vi "Mapping v10.4.0.vi"(5 "Simulate Spectra":bool, 7 "Simulate Drive":bool, 11 "Input Parameters":T9={"CCD3000 Connection"={"Comm Interface"=1, "BUS"=0, "Address"=5, "Com Port"=1}, "Drive Connection Settings"={"Objective GPIB-Port"=4, "Stage GPIB-Port"=4, "Drive Selector"=0, "Drive Velocity (V/s)"=5.0}, "ITC503 Current Values"={"ITC503 Heater"=0.0, "ITC503 Temperature"=0.0, "ITC503 P"=0.0, "ITC503 I"=0.0, "ITC503 D"=0.0, "ITC503 Setpoint"=0.0, "ITC503 Gradient"=0.0, "ITC503 Heater Auto"=FALSE, "ITC503 PID Auto"=FALSE}, "Wavelengths (nm)"=[], "Drive Current Values"={"Voltages"={"Drive X Voltage"=0.0, "Drive Y Voltage"=0.0, "Drive Z Voltage"=0.0}, "Position"={"Drive X Position"=0.0, "Drive Y Position"=0.0, "Drive Z Position"=0.0}}, "iHR Current Values"={"iHR 550 Front Entrance"=0.0, "iHR550 Side Exit"=0.0, "iHR550 Wavelength"=897.9988, "iHR550 Exit Mirror"=2, "iHR550 Grating"="1", "Grating Index"=1}, "Spectra Settings"={"Integration Time"=1.0, "Repetitions"=1, "Mapping Spectra"=TRUE}, "CCD3500 Temperature"=0.0, "Simulate Drive"=FALSE, "Simulate Spectra"=FALSE} {"CCD3500 Temperature" min=10.0 max=160.0 step=0.1 format="%.1f"; "Spectra Settings"."Repetitions" min=1 max=100 step=1; "Spectra Settings"."Integration Time" min=0.5 max=6000.0 step=1.0 format="%.1f"; "iHR Current Values"."iHR550 Exit Mirror" items=["EntranceMirror", "ExitMirror", "Front", "Side"]; "Drive Current Values"."Position"."Drive Z Position" min=-273.0 max=300000.0 step=0.0001 format="%.1f"; "Drive Current Values"."Position"."Drive Y Position" min=-273.0 max=300000.0 step=0.0001 format="%.1f"; "Drive Current Values"."Position"."Drive X Position" min=-273.0 max=300000.0 step=0.0001 format="%.1f"; "Drive Current Values"."Voltages"."Drive Z Voltage" min=-273.0 max=300000.0 step=0.0001 format="%.1f"; "Drive Current Values"."Voltages"."Drive Y Voltage" min=-273.0 max=300000.0 step=0.0001 format="%.1f"; "Drive Current Values"."Voltages"."Drive X Voltage" min=-273.0 max=300000.0 step=0.0001 format="%.1f"; "ITC503 Current Values"."ITC503 Gradient" format="%.2f"; "ITC503 Current Values"."ITC503 Setpoint" min=-273.0 max=300000.0 step=0.0001 format="%.1f"; "ITC503 Current Values"."ITC503 I" format="%_1f"; "ITC503 Current Values"."ITC503 P" format="%_1f"; "ITC503 Current Values"."ITC503 Temperature" min=0.0 max=1645.0 step=1e-05 format="%.2f"; "ITC503 Current Values"."ITC503 Heater" min=0.0 max=100.0 step=0.01 scale=0.0..100.0; "Drive Connection Settings"."Drive Velocity (V/s)" min=10.0 max=160.0 step=0.1 format="%.1f"; "Drive Connection Settings"."Drive Selector" items=["Obj.", "Stage"]; "Drive Connection Settings"."Stage GPIB-Port" min=1 max=20 step=1 format="%#.0f"; "Drive Connection Settings"."Objective GPIB-Port" min=1 max=20 step=1 format="%#.0f"; "CCD3000 Connection"."Comm Interface" items=["RS 232", "GPIB"]}) -> ()   [LabVIEW 2010]
uses:
  ESA-C/TypeDefs/ESA-C Connection Settings.ctl
  TypeDefs/Mapping Spectra Params.ctl
  TypeDefs/Mapping Drive Params.ctl
  ESA-C/TypeDefs/ESA-C Set Positions.ctl
  ESA-C/TypeDefs/ESA-C Current Values.ctl
  iHR550/TypeDefs/iHR Current Values.ctl
  ITC503/TypeDefs/ITC503 Current Values.ctl
  drivers/Horiba Spectrum One 3000V/Lib/CCD_command.llb/Comm Params.ctl
  <vilib>/Utility/miscctls.llb/LVPointTypeDef.ctl
  Global Variables.vi
panel:
  out "AutoClose":bool
  out "ITC503 Temperature":dbl caption="Sample (K)" min=10.0 max=160.0 step=0.1 format="%.1f"
  out "CCD3500 Temperature":dbl caption="CCD (°C)" min=10.0 max=160.0 step=0.1 format="%.1f"
  in  "CCD3000 Current Rep.":string="0/0"
  in  "Pause":bool
  out "Current Position":T1 {"Position"."Drive Z Position" min=-273.0 max=300000.0 step=0.0001 format="%.1f"; "Position"."Drive Y Position" min=-273.0 max=300000.0 step=0.0001 format="%.1f"; "Position"."Drive X Position" min=-273.0 max=300000.0 step=0.0001 format="%.1f"; "Voltages"."Drive Z Voltage" min=-273.0 max=300000.0 step=0.0001 format="%.1f"; "Voltages"."Drive Y Voltage" min=-273.0 max=300000.0 step=0.0001 format="%.1f"; "Voltages"."Drive X Voltage" min=-273.0 max=300000.0 step=0.0001 format="%.1f"}
  out "Target Position":T2={"Drive X Set"=10.0, "Drive Y Set"=10.0, "Drive Z Set"=10.0} {"Drive X Set" min=10.0 max=160.0 step=0.1 format="%.1f"; "Drive Z Set" min=10.0 max=160.0 step=0.1 format="%.1f"; "Drive Y Set" min=10.0 max=160.0 step=0.1 format="%.1f"}
  out "Progress":u8(slide) max=10 scale=0.0..100.0
  out "Objective Running":bool caption="Obj."
  out "CCD Running":bool caption="CCD"
  in  "Save Map":bool
  in  "Spectra Params":T3={"Integration Time"=10.0, "Repetitions"=10, "Mapping Spectra"=TRUE} {"Repetitions" min=1 max=100 step=1; "Integration Time" min=0.5 max=6000.0 step=1.0 format="%.1f"}
  in  "Drive Settings":T4={"Objective GPIB-Port"=4, "Stage GPIB-Port"=4, "Drive Selector"=0, "Drive Velocity (V/s)"=5.0} {"Drive Velocity (V/s)" min=10.0 max=160.0 step=0.1 format="%.1f"; "Drive Selector" items=["Obj.", "Stage"]; "Stage GPIB-Port" min=1 max=20 step=1 format="%#.0f"; "Objective GPIB-Port" min=1 max=20 step=1 format="%#.0f"}
  in  "Z Position":dbl caption="Z (µm)" min=0.0 max=100.0 step=0.1 format="%.1f"
  in  "Mapping Params":T5={"X Start Position"=0.0, "X Stop Position"=10.0, "Y Start Position"=0.0, "Y Stop Position"=10.0, "Step Size"=1.0} {"Step Size" min=0.1 max=30.0 step=0.1 format="%.1f"; "Y Stop Position" min=0.0 max=30.0 step=0.1 format="%.1f"; "Y Start Position" min=0.0 max=30.0 step=0.1 format="%.1f"; "X Stop Position" min=0.0 max=30.0 step=0.1 format="%.1f"; "X Start Position" min=0.0 max=30.0 step=0.1 format="%.1f"}
  in  "Exit":bool
  out "Measuring":bool
  in  "Start":bool
  out "Filename":string
  out "Full Data":dbl[][](array[numeric])
  in  "CCD3500V Connection":T10={"Comm Interface"=1, "BUS"=0, "Address"=5, "Com Port"=0}
  out "Live Data":dbl[][](array[numeric])
  in  "ITC503 Current Values":T7 {"ITC503 Gradient" format="%.2f"; "ITC503 Setpoint" min=-273.0 max=300000.0 step=0.0001 format="%.1f"; "ITC503 I" format="%_1f"; "ITC503 P" format="%_1f"; "ITC503 Temperature" min=0.0 max=1645.0 step=1e-05 format="%.2f"; "ITC503 Heater" min=0.0 max=100.0 step=0.01 scale=0.0..100.0}
  in  "iHR Current Values":T8={"iHR 550 Front Entrance"=0.0, "iHR550 Side Exit"=0.0, "iHR550 Wavelength"=897.9988, "iHR550 Exit Mirror"=2, "iHR550 Grating"="1", "Grating Index"=1} {"iHR550 Exit Mirror" items=["EntranceMirror", "ExitMirror", "Front", "Side"]}
  in  "Wavelengths (nm)":dbl[](array[numeric])
  # "Status"
  # "Active"
  # "Target"
  # "Current"
  # "Parameters"
  # "Spectral"
  # "Spectral / Video Mapping"
  # "Mapping"
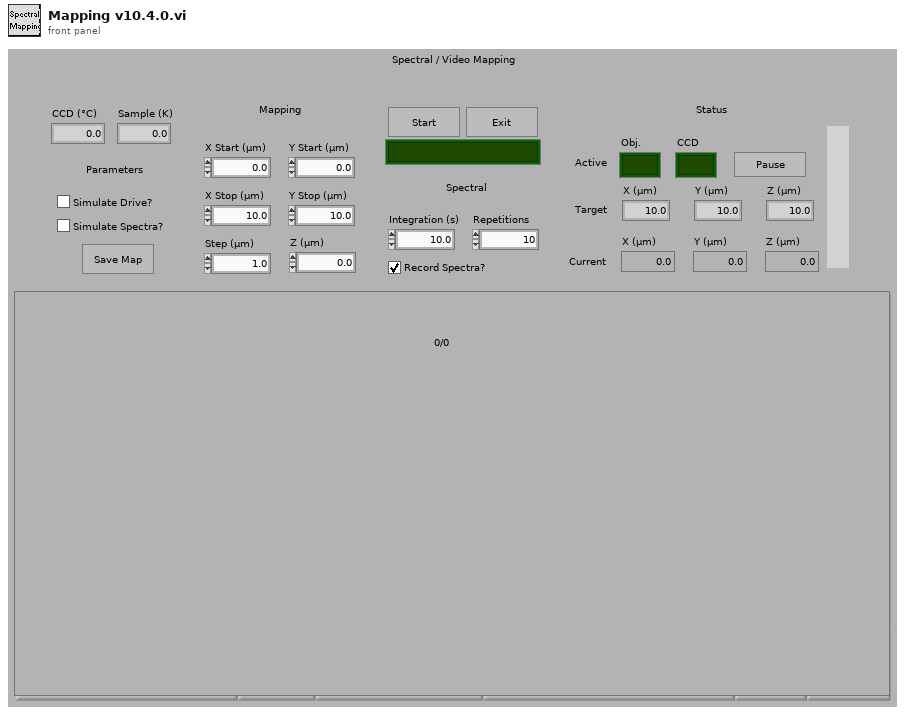
[diagram p1: front panel]
types:
  T1 = typedef "ESA-C Current Values.ctl" = cluster{"Voltages":cluster{"Drive X Voltage":dbl, "Drive Y Voltage":dbl, "Drive Z Voltage":dbl}, "Position":cluster{"Drive X Position":dbl, "Drive Y Position":dbl, "Drive Z Position":dbl}}
  T2 = typedef "ESA-C Set Positions.ctl" = cluster{"Drive X Set":dbl, "Drive Y Set":dbl, "Drive Z Set":dbl}
  T3 = typedef "Mapping Spectra Params.ctl" = cluster{"Integration Time":dbl, "Repetitions":u16, "Mapping Spectra":bool}
  T4 = typedef "ESA-C Connection Settings.ctl" = cluster{"Objective GPIB-Port":i32, "Stage GPIB-Port":i32, "Drive Selector":u16, "Drive Velocity (V/s)":dbl}
  T5 = typedef "Mapping Drive Params.ctl" = cluster{"X Start Position":dbl, "X Stop Position":dbl, "Y Start Position":dbl, "Y Stop Position":dbl, "Step Size":dbl}
  T6 = typedef "Comm Params.ctl" = cluster{"Comm Interface":u16, "BUS":i16, "Address":i16, "Com Port":i32}
  T7 = typedef "ITC503 Current Values.ctl" = cluster{"ITC503 Heater":dbl, "ITC503 Temperature":dbl, "ITC503 P":dbl, "ITC503 I":dbl, "ITC503 D":dbl, "ITC503 Setpoint":dbl, "ITC503 Gradient":dbl, "ITC503 Heater Auto":bool, "ITC503 PID Auto":bool}
  T8 = typedef "iHR Current Values.ctl" = cluster{"iHR 550 Front Entrance":dbl, "iHR550 Side Exit":dbl, "iHR550 Wavelength":dbl, "iHR550 Exit Mirror":i32, "iHR550 Grating":string, "Grating Index":i32}
  T9 = cluster{"CCD3000 Connection":T6, "Drive Connection Settings":T4, "ITC503 Current Values":T7, "Wavelengths (nm)":dbl[], "Drive Current Values":T1, "iHR Current Values":T8, "Spectra Settings":T3, "CCD3500 Temperature":dbl, "Simulate Drive":bool, "Simulate Spectra":bool}
  T10 = cluster{"Comm Interface":u16, "BUS":i16, "Address":i16, "Com Port":i32}
  T11 = cluster{"CCD3000 Connection":T6, "Drive Connection Settings":T4, "ITC503 Current Values":T7, "Wavelengths (nm)":dbl[], "Drive Current Values":T1, "iHR Current Values":T8, "Spectra Settings":T3, "CCD3500 Temperature":dbl, "Simulate Drive 2":bool, "Simulate Spectra 2":bool}
  T12 = typedef "LVPointTypeDef.ctl" = cluster{"Horizontal":i16, "Vertical":i16}
  T13 = typedef "NPC3SG Set Positions.ctl" = cluster{"Drive X Set":dbl, "Drive Y Set":dbl, "Drive Z Set":dbl}
  T14 = cluster{"Intensities":dbl[], "Wavelengths":dbl[]}[]
  T15 = cluster{"Intensities":dbl[], "Wavelengths":dbl[]}
  T16 = enum32{"invalid app kind", "Development System", "Run Time System", "Student Edition", "Embedded LabVIEW", "Evaluation", "Custom"}
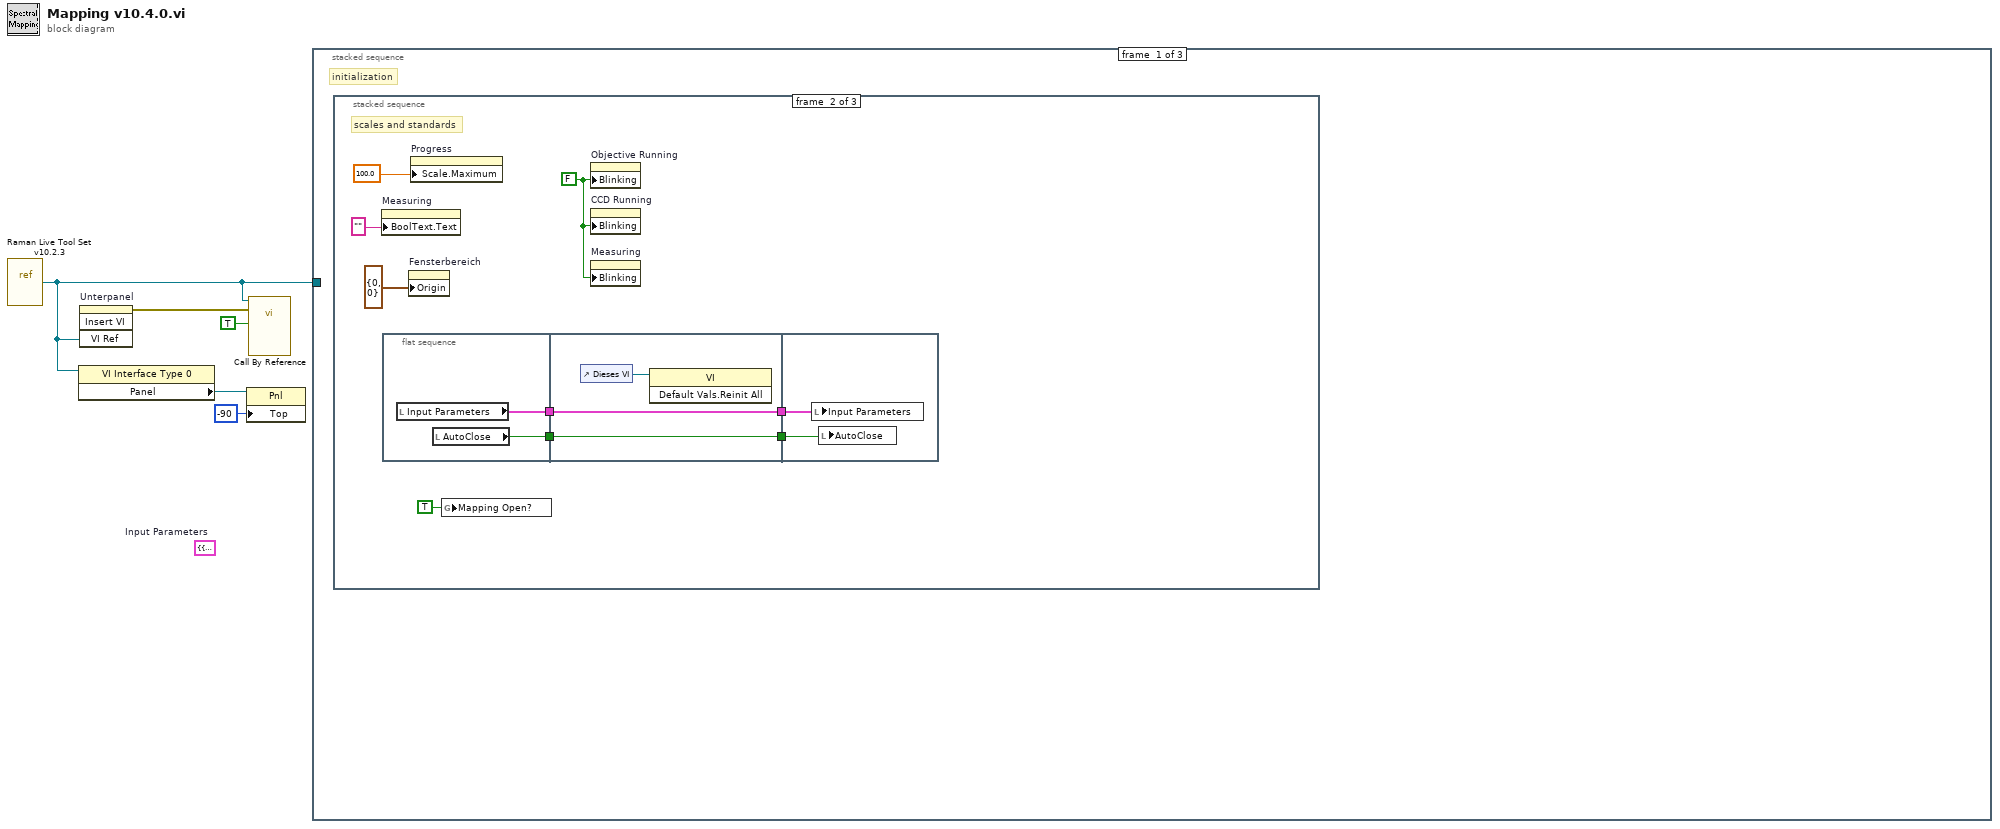
[diagram p0: block diagram]
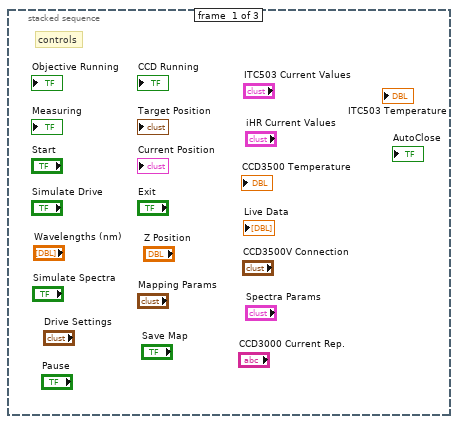
[diagram p2: hidden frame]
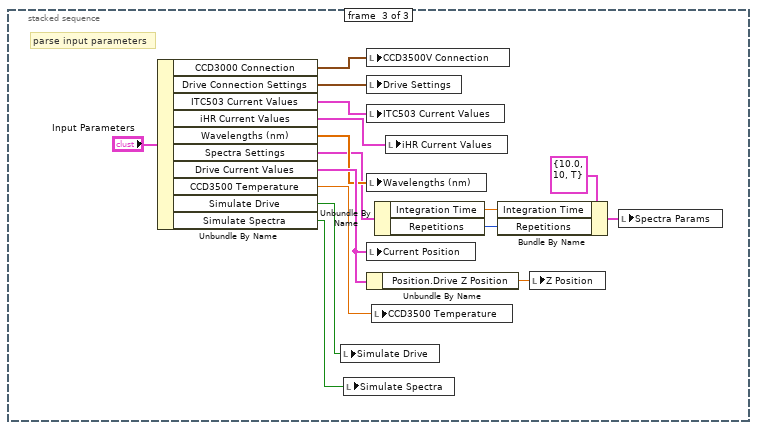
[diagram p3: hidden frame]
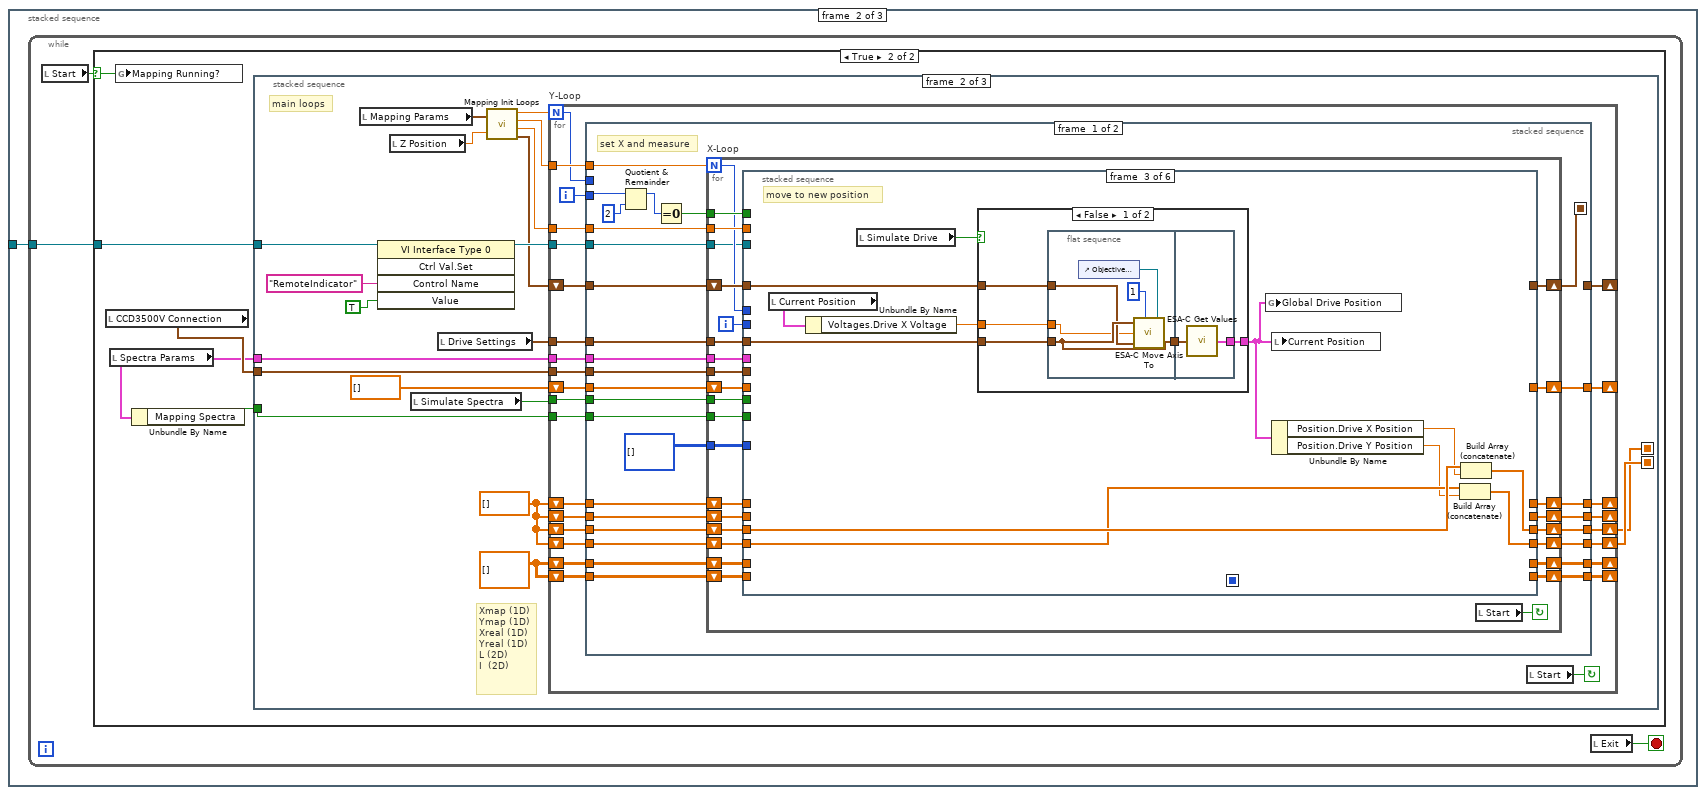
[diagram p4: hidden frame]
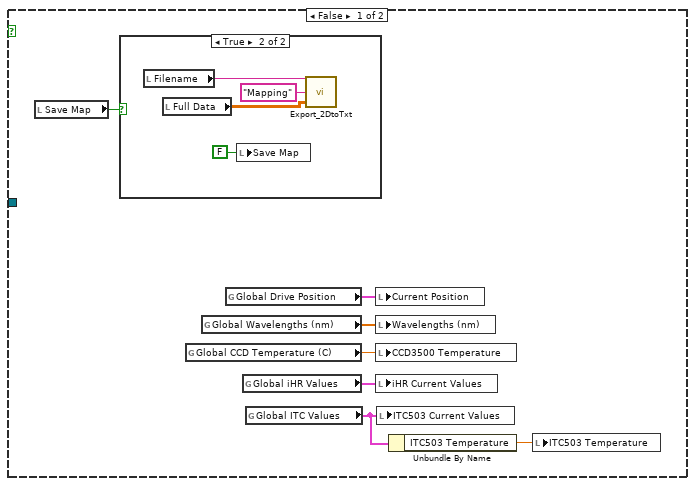
[diagram p5: hidden frame]
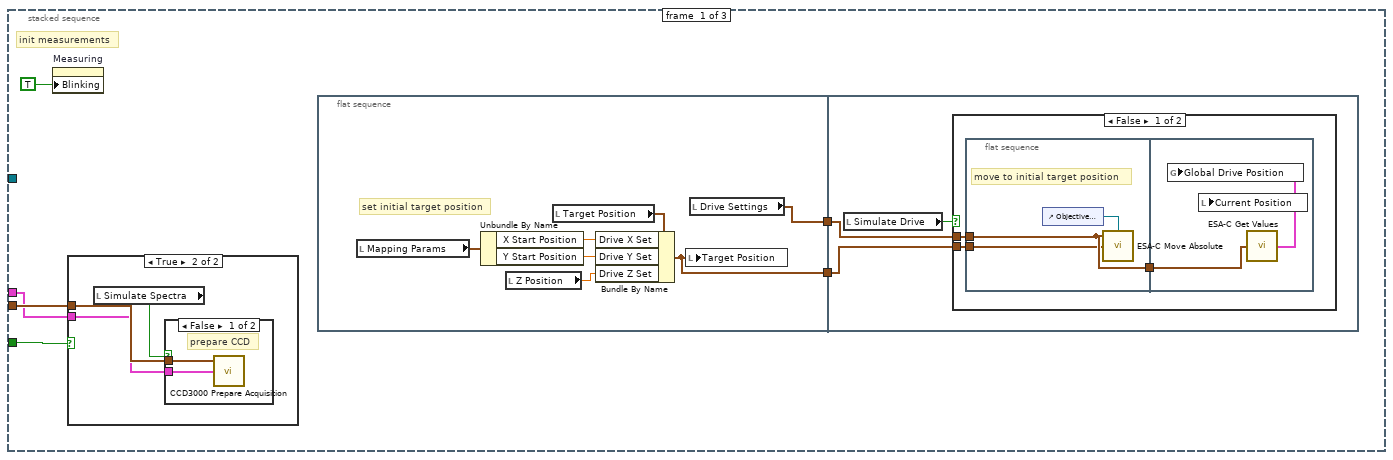
[diagram p7: hidden frame]
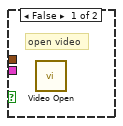
[diagram p9: hidden frame]
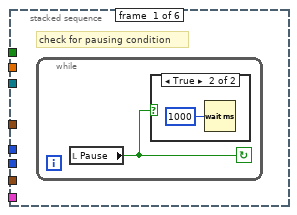
[diagram p11: hidden frame]
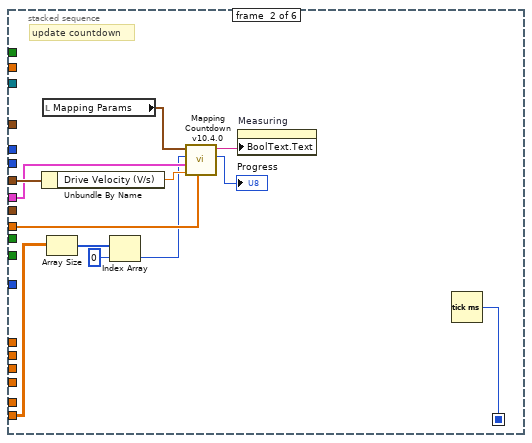
[diagram p13: hidden frame]
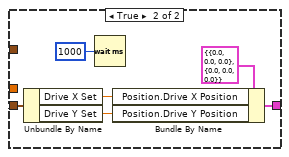
[diagram p14: hidden frame]
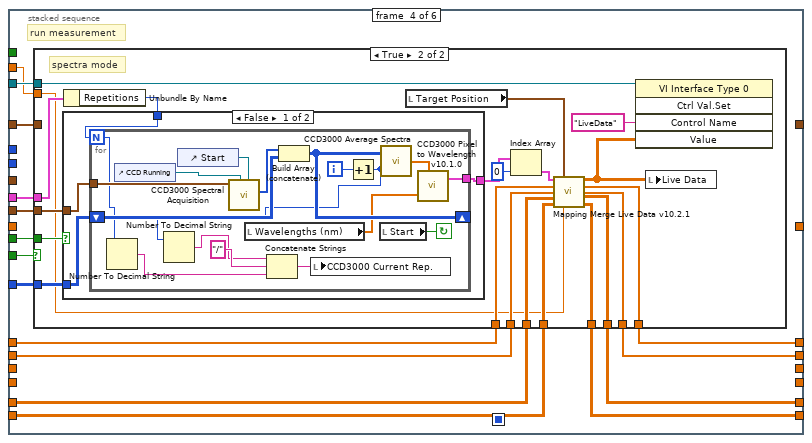
[diagram p15: hidden frame]
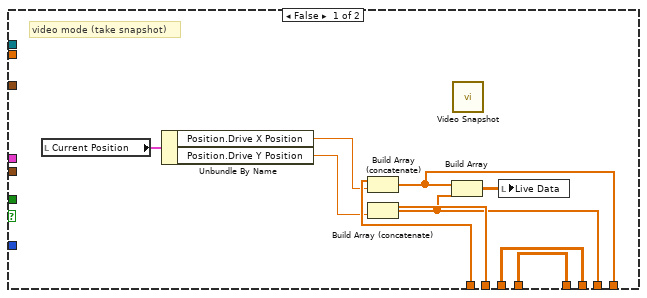
[diagram p16: hidden frame]
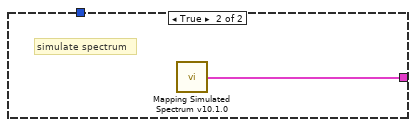
[diagram p17: hidden frame]
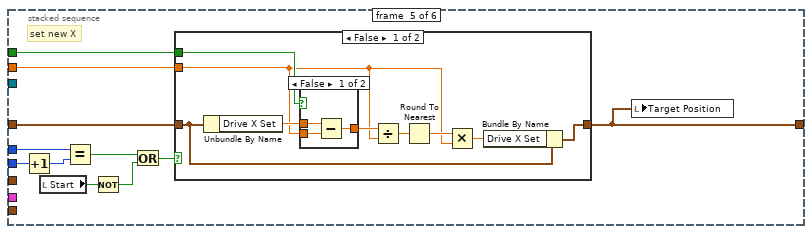
[diagram p18: hidden frame]
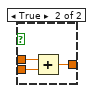
[diagram p19: hidden frame]
diagram:
  (unwired) T11 {"CCD3000 Connection"={"Comm Interface"=1, "BUS"=0, "Address"=5, "Com Port"=1}, "Drive Connection Settings"={"Objective GPIB-Port"=4, "Stage GPIB-Port"=4, "Drive Selector"=0, "Drive Velocity (V/s)"=5.0}, "ITC503 Current Values"={"ITC503 Heater"=0.0, "ITC503 Temperature"=0.0, "ITC503 P"=0.0, "ITC503 I"=0.0, "ITC503 D"=0.0, "ITC503 Setpoint"=0.0, "ITC503 Gradient"=0.0, "ITC503 Heater Auto"=FALSE, "ITC503 PID Auto"=FALSE}, "Wavelengths (nm)"=[], "Drive Current Values"={"Voltages"={"Drive X Voltage"=0.0, "Drive Y Voltage"=0.0, "Drive Z Voltage"=0.0}, "Position"={"Drive X Position"=0.0, "Drive Y Position"=0.0, "Drive Z Position"=0.0}}, "iHR Current Values"={"iHR 550 Front Entrance"=0.0, "iHR550 Side Exit"=0.0, "iHR550 Wavelength"=897.9988, "iHR550 Exit Mirror"=2, "iHR550 Grating"="1", "Grating Index"=1}, "Spectra Settings"={"Integration Time"=1.0, "Repetitions"=1, "Mapping Spectra"=TRUE}, "CCD3500 Temperature"=0.0, "Simulate Drive 2"=FALSE, "Simulate Spectra 2"=FALSE}  # Input Parameters
  n1 = vi-ref "Raman Live Tool Set v10.2.3.vi"() -> (w3:refnum<vi>)
  n2 = property class="VI Interface Type 0"(reference=w3) -> ("Panel"=w2:refnum<vi>)  [unwired: 1 in, 2 out]
  n3 = invoke on="Unterpanel" class="Unterpanel" method="Insert VI"("VI Ref"=w3) -> (error out=w5:errorcluster)  [unwired: 3 in, 3 out]
  n4 = property class="Pnl"(reference=w2, "Top"=-90 ("Position:Oben")) -> ()  [unwired: 1 in, 2 out]
  n5 = call-by-ref "?"(reference=w3, error in=w5, "RemoteIndicator"=TRUE) -> ()  [unwired: 3 in, 2 out]
  n6 = stacked-sequence {
    tunnel: w3 -> [_ w38 w394]
    frame #0 {
      # "initialization"
      n7 = stacked-sequence {
        frame #0 {
          # "controls"
        }
        frame #1 {
          w12 = FALSE ("Blinkend")
          # "scales and standards"
          n8 = property on="Measuring" class="Bool (strict)"("BoolText.Text"="" ("Boolescher Text.Text")) -> ()  [unwired: 2 in, 2 out]
          n9 = flat-sequence {
            tunnel: [w16] -> w9
            tunnel: [w15] -> w6
            tunnel: [w18] -> w10
            tunnel: w9 -> [w18]
            tunnel: [w17] -> w7
            tunnel: w6 -> [w17]
            tunnel: w10 -> [w21]
            tunnel: w7 -> [w20]
            frame #0 {
              n10 = local read "Input Parameters"() -> (w16:T9)
              n11 = local read "AutoClose"() -> (w15:bool)
            }
            frame #1 {
              n12 = control-ref of="Dieses VI"() -> (w19:refnum<vi>)
              n13 = invoke class="VI" method="Default Vals.Reinit All"(reference=w19) -> ()  [unwired: 2 in, 3 out]
            }
            frame #2 {
              n14 = local write "Input Parameters"(w21) -> ()
              n15 = local write "AutoClose"(w20) -> ()
            }
          }
          n16 = property on="Fensterbereich" class="Pane"("Origin"=T12 {"Horizontal"=0, "Vertical"=0}) -> ()  [unwired: 2 in, 2 out]
          n17 = property on="Progress" class="Slide (strict)"("Scale.Maximum"=100.0 ("Skalierung.Bereich:Maximum")) -> ()  [unwired: 2 in, 2 out]
          n18 = global write "Global Variables.vi" "Mapping Open?"(TRUE ("Mapping Open?")) -> ()
          n19 = property on="Objective Running" class="Bool (strict)"("Blinking"=w12) -> ()  [unwired: 2 in, 2 out]
          n20 = property on="CCD Running" class="Bool (strict)"("Blinking"=w12) -> ()  [unwired: 2 in, 2 out]
          n21 = property on="Measuring" class="Bool (strict)"("Blinking"=w12) -> ()  [unwired: 2 in, 2 out]
        }
        frame #2 {
          # "parse input parameters"
          n22 = Unbundle By Name("Input Parameters") -> ("CCD3000 Connection"=w34:T6, "Drive Connection Settings"=w35:T4, "ITC503 Current Values"=w36:T7, "iHR Current Values"=w25:T8, "Wavelengths (nm)"=w33:dbl[], "Spectra Settings"=w31:T3, "Drive Current Values"=w37:T1, "CCD3500 Temperature"=w26:dbl, "Simulate Drive"=w23:bool, "Simulate Spectra"=w22:bool)
          n23 = local write "Simulate Drive"(w23) -> ()
          n24 = local write "Simulate Spectra"(w22) -> ()
          n25 = local write "CCD3500V Connection"(w34) -> ()
          n26 = local write "Drive Settings"(w35) -> ()
          n27 = local write "ITC503 Current Values"(w36) -> ()
          n28 = local write "Wavelengths (nm)"(w33) -> ()
          n29 = local write "Current Position"(w37) -> ()
          n30 = Unbundle By Name(w37) -> ("Position.Drive Z Position"=w32:dbl)
          n31 = local write "CCD3500 Temperature"(w26) -> ()
          n32 = Unbundle By Name(w31) -> ("Integration Time"=w29:dbl, "Repetitions"=w28:u16)
          n33 = local write "iHR Current Values"(w25) -> ()
          n34 = Bundle By Name(cluster=T3 {"Integration Time"=10.0, "Repetitions"=10, "Mapping Spectra"=TRUE} ("Mapping Spectra Settings"), "Integration Time"=w29, "Repetitions"=w28) -> (w27:T3)
          n35 = local write "Z Position"(w32) -> ()
          n36 = local write "Spectra Params"(w27) -> ()
        }
      }
    }
    frame #1 {
      n37 = while {
        tunnel: w38 -> [w41]
        stop <- w40 stop-if-true
        n38 = local read "Start"() -> (w39:bool)
        n39 = case shown="True" w39 {
          selector: w39 -> [_ w53]
          tunnel: w41 -> [_ w57]
          frame False {
            n40 = local read "Save Map"() -> (w48:bool)
            n41 = case shown="True" w48 {
              frame False {
              }
              frame True {
                n42 = local read "Filename"() -> (w51:string)
                n43 = local read "Full Data"() -> (w49:dbl[][])
                n44 = local write "Save Map"(FALSE ("Save Map")) -> ()
                n45 = call "Export_2DtoTxt.vi"("Data (2D)"=w49, "Export Type"="Mapping", "Filename"=w51) -> ()  [unwired: 3 in]
              }
            }
            n46 = global read "Global Variables.vi" "Global CCD Temperature (C)"() -> (w47:dbl)
            n47 = global read "Global Variables.vi" "Global Wavelengths (nm)"() -> (w45:dbl[])
            n48 = global read "Global Variables.vi" "Global Drive Position"() -> (w46:T1)
            n49 = global read "Global Variables.vi" "Global iHR Values"() -> (w44:T8)
            n50 = global read "Global Variables.vi" "Global ITC Values"() -> (w43:T7)
            n51 = local write "Current Position"(w46) -> ()
            n52 = local write "Wavelengths (nm)"(w45) -> ()
            n53 = local write "CCD3500 Temperature"(w47) -> ()
            n54 = local write "iHR Current Values"(w44) -> ()
            n55 = local write "ITC503 Current Values"(w43) -> ()
            n56 = Unbundle By Name(w43) -> ("ITC503 Temperature"=w42:dbl)
            n57 = local write "ITC503 Temperature"(w42) -> ()
          }
          frame True {
            n58 = local read "CCD3500V Connection"() -> (w55:T10)
            n59 = local read "Spectra Params"() -> (w54:T3)
            n60 = global write "Global Variables.vi" "Mapping Running?"(w53) -> ()
            n61 = Unbundle By Name(w54) -> ("Mapping Spectra"=w56:bool)
            n62 = stacked-sequence {
              seq-local: [_ w87 _] -> [_ _ w373]
              seq-local: [_ w88 _] -> [_ _ w372]
              tunnel: w57 -> [_ w98 _]
              tunnel: w56 -> [w62 w97 w374]
              tunnel: w54 -> [w60 w95 _]
              tunnel: w55 -> [w61 w94 _]
              frame #0 {
                # "init measurements"
                n63 = property on="Measuring" class="Bool (strict)"("Blinking"=TRUE ("Blinkend")) -> ()  [unwired: 2 in, 2 out]
                n64 = case shown="True" w62 {
                  tunnel: w61 -> [_ w84]
                  tunnel: w60 -> [_ w83]
                  frame False {
                    # "open video"
                    n65 = call "Video Open.vi"() -> ()  [unwired: 11 in, 1 out]
                  }
                  frame True {
                    n66 = local read "Simulate Spectra"() -> (w82:bool)
                    n67 = case shown="False" w82 {
                      tunnel: w84 -> [w86 _]
                      tunnel: w83 -> [w85 _]
                      frame False {
                        # "prepare CCD"
                        n68 = call "CCD3000 Prepare Acquisition.vi"("Mapping Spectra Settings"=w85, "Comm Params"=w86) -> ()  [unwired: 4 in]
                      }
                      frame True {
                      }
                    }
                  }
                }
                n69 = flat-sequence {
                  tunnel: [w65] -> w59
                  tunnel: [w64] -> w58
                  tunnel: w59 -> [w71]
                  tunnel: w58 -> [w72]
                  frame #0 {
                    # "set initial target position"
                    n70 = local read "Mapping Params"() -> (w70:T5)
                    n71 = Unbundle By Name(w70) -> ("X Start Position"=w68:dbl, "Y Start Position"=w67:dbl)
                    n72 = local read "Z Position"() -> (w66:dbl)
                    n73 = local read "Target Position"() -> (w69:T2)
                    n74 = Bundle By Name(cluster=w69, "Drive X Set"=w68, "Drive Y Set"=w67, "Drive Z Set"=w66) -> (w65:T2)
                    n75 = local write "Target Position"(w65) -> ()
                    n76 = local read "Drive Settings"() -> (w64:T4)
                  }
                  frame #1 {
                    n77 = local read "Simulate Drive"() -> (w73:bool)
                    n78 = case shown="False" w73 {
                      tunnel: w72 -> [w76 _]
                      tunnel: w71 -> [w74 _]
                      frame False {
                        n79 = flat-sequence {
                          tunnel: w76 -> [w78]
                          tunnel: [w78] -> w75
                          tunnel: w74 -> [w77]
                          tunnel: w75 -> [w81]
                          frame #0 {
                            # "move to initial target position"
                            n80 = control-ref of="Objective Running"() -> (w79:refnum<vi>)
                            n81 = call "ESA-C Move Absolute.vi"("Running"=w79, "Drive New Abs. Positions"=w77, "Drive Connection Settings"=w78) -> ()  [unwired: 2 in]
                          }
                          frame #1 {
                            n82 = call "ESA-C Get Values.vi"("Drive Connection Settings"=w81) -> ("Drive Current Values"=w80:T1)
                            n83 = global write "Global Variables.vi" "Global Drive Position"(w80) -> ()
                            n84 = local write "Current Position"(w80) -> ()
                          }
                        }
                      }
                      frame True {
                      }
                    }
                  }
                }
              }
              frame #1 {
                w106 = dbl[][] []
                w89 = dbl[] []
                # "main loops"
                # "Xmap (1D)\nYmap (1D)\nXreal (1D)\nYreal (1D)\nL (2D)\nI  (2D)"
                n85 = local read "Mapping Params"() -> (w92:T5)
                n86 = invoke class="VI Interface Type 0" method="Ctrl Val.Set"(reference=w98, "Control Name"="RemoteIndicator" ("Elementname"), "Value"=TRUE) -> (reference out=w100:refnum<vi>)  [unwired: 2 in, 4 out]
                n87 = local read "Z Position"() -> (w91:dbl)
                n88 = local read "Simulate Spectra"() -> (w90:bool)
                n89 = local read "Drive Settings"() -> (w93:T4)
                n90 = call "Mapping Init Loops.vi"("Z Position"=w91, "Mapping Params"=w92) -> ("Start Positions"=w99:T13, "Step Size"=w101:dbl, "X Steps"=w102:dbl, "Y Steps"=w103:dbl)
                n91 = for "Y-Loop" {
                  N: w103 -> [w119]
                  tunnel: w102 -> [w132]
                  tunnel: w101 -> [w131]
                  shift-right: [w117] -> _
                  shift-left: w99 -> [w118]
                  shift-right: [w123] -> _
                  shift-left: w106 -> [w127]
                  shift-right: [w124] -> _
                  shift-left: w106 -> [w128]
                  shift-right: [w126] -> _
                  shift-left: w89 -> [w130]
                  shift-right: [w125] -> _
                  shift-left: w89 -> [w129]
                  tunnel: w100 -> [w121]
                  tunnel: w90 -> [w120]
                  tunnel: w93 -> [w116]
                  tunnel: w97 -> [w115]
                  tunnel: w95 -> [w114]
                  shift-right: [w112] -> _
                  shift-left: dbl[] [] -> [w113]
                  tunnel: w94 -> [w111]
                  shift-right: [w108] -> w88
                  shift-left: w89 -> [w109]
                  shift-right: [w107] -> w87
                  shift-left: w89 -> [w110]
                  i -> [w122]
                  stop <- w133 continue-if-true
                  n92 = stacked-sequence {
                    seq-local: [w147 _] -> [_ w345]
                    tunnel: w132 -> [w162 _]
                    tunnel: w131 -> [w161 w346]
                    tunnel: w130 -> [w160 _]
                    tunnel: w129 -> [w159 _]
                    tunnel: w128 -> [w158 _]
                    tunnel: w127 -> [w134 _]
                    tunnel: [w157 _] -> w126
                    tunnel: [w156 _] -> w125
                    tunnel: [w155 _] -> w124
                    tunnel: [w154 _] -> w123
                    tunnel: w122 -> [w151 w349]
                    tunnel: w121 -> [w149 _]
                    tunnel: w120 -> [w148 _]
                    tunnel: w119 -> [_ w347]
                    tunnel: w118 -> [w146 _]
                    tunnel: [_ w343] -> w117
                    tunnel: w116 -> [w145 w344]
                    tunnel: w115 -> [w144 _]
                    tunnel: w114 -> [w143 _]
                    tunnel: w113 -> [w142 _]
                    tunnel: [w141 _] -> w112
                    tunnel: w111 -> [w140 _]
                    tunnel: w110 -> [w138 _]
                    tunnel: w109 -> [w137 _]
                    tunnel: [w136 _] -> w108
                    tunnel: [w135 _] -> w107
                    frame #0 {
                      # "set X and measure"
                      n93 = Quotient & Remainder(x=w151, y=2) -> (x-y*floor(x/y)=w152:i32)  [unwired: 1 out]
                      n94 = Equal To 0?(x=w152) -> (x = 0?=w150:bool)
                      n95 = for "X-Loop" {
                        N: w162 -> [w176]
                        tunnel: w161 -> [w188]
                        shift-right: [w187] -> w147
                        shift-left: w146 -> [w189]
                        shift-right: [w182] -> w157
                        shift-left: w160 -> [w186]
                        shift-right: [w181] -> w156
                        shift-left: w159 -> [w185]
                        shift-right: [w179] -> w155
                        shift-left: w158 -> [w184]
                        shift-right: [w180] -> w154
                        shift-left: w134 -> [w183]
                        tunnel: w150 -> [w178]
                        tunnel: w149 -> [w175]
                        tunnel: w148 -> [w174]
                        tunnel: w145 -> [w173]
                        tunnel: w144 -> [w172]
                        tunnel: w143 -> [w171]
                        shift-right: [w170] -> w141
                        shift-left: w142 -> [w169]
                        tunnel: w140 -> [w168]
                        tunnel: u16[][] [] -> [w167]
                        shift-right: [w163] -> w135
                        shift-left: w138 -> [w166]
                        shift-right: [w164] -> w136
                        shift-left: w137 -> [w165]
                        i -> [w177]
                        stop <- w190 continue-if-true
                        n96 = stacked-sequence {
                          seq-local: [_ w197 _ _ _ _] -> [_ _ _ _ _ w334]
                          tunnel: w189 -> [_ _ w216 w250 w311 _]
                          tunnel: w188 -> [_ _ _ w235 w309 _]
                          tunnel: [_ _ _ _ w308 _] -> w187
                          tunnel: w186 -> [_ _ _ w249 _ _]
                          tunnel: w185 -> [_ _ _ w248 _ _]
                          tunnel: w184 -> [_ _ _ w246 _ _]
                          tunnel: w183 -> [_ w196 _ w247 _ _]
                          tunnel: [_ _ _ w245 _ _] -> w182
                          tunnel: [_ _ _ w244 _ _] -> w181
                          tunnel: [_ _ _ w243 _ _] -> w180
                          tunnel: [_ _ _ w242 _ _] -> w179
                          tunnel: w178 -> [_ _ _ _ w310 _]
                          tunnel: w177 -> [_ _ _ _ w314 _]
                          tunnel: w176 -> [_ _ _ _ w312 _]
                          tunnel: w175 -> [_ _ _ w241 _ _]
                          tunnel: w174 -> [_ _ _ w240 _ _]
                          tunnel: w173 -> [_ w200 w214 _ _ _]
                          tunnel: w172 -> [_ _ _ w239 _ _]
                          tunnel: w171 -> [_ w199 _ w237 _ _]
                          tunnel: [_ _ _ _ _ w331] -> w170
                          tunnel: w169 -> [_ w198 _ _ _ w333]
                          tunnel: w168 -> [_ _ _ w238 _ _]
                          tunnel: w167 -> [_ _ _ w236 _ _]
                          tunnel: w166 -> [_ _ w211 _ _ _]
                          tunnel: w165 -> [_ _ w210 _ _ _]
                          tunnel: [_ _ w207 _ _ _] -> w164
                          tunnel: [_ _ w206 _ _ _] -> w163
                          frame #0 {
                            # "check for pausing condition"
                            n97 = while {
                              stop <- w191 continue-if-true
                              n98 = local read "Pause"() -> (w191:bool)
                              n99 = case shown="True" w191 {
                                frame False {
                                }
                                frame True {
                                n100 = Wait (ms)(milliseconds to wait=u32 1000) -> ()  [unwired: 1 out]
                                }
                              }
                            }
                          }
                          frame #1 {
                            # "update countdown"
                            n101 = Unbundle By Name(w200) -> ("Drive Velocity (V/s)"=w201:dbl)
                            n102 = local read "Mapping Params"() -> (w204:T5)
                            n103 = Array Size(array=w196) -> (size(s)=w195:i32[])
                            n104 = Index Array(array=w195, index=0) -> (element=w193:i32)
                            n105 = call "Mapping Countdown v10.4.0.vi"("Execution Times (s)"=w198, "Drive Velocity"=w201, "Mapping Spectra Settings"=w199, "Ready Steps"=w193, "Mapping Drive Parameters"=w204) -> ("Progress"=→"Progress":i16, "Time String"=w202:string)  [unwired: 5 in]
                            n106 = property on="Measuring" class="Bool (strict)"("BoolText.Text"=w202) -> ()  [unwired: 2 in, 2 out]
                            n107 = Tick Count (ms)() -> (millisecond timer value=w197:u32)
                          }
                          frame #2 {
                            # "move to new position"
                            n108 = local read "Current Position"() -> (w213:T1)
                            n109 = Unbundle By Name(w213) -> ("Voltages.Drive X Voltage"=w212:dbl)
                            n110 = local read "Simulate Drive"() -> (w215:bool)
                            n111 = case shown="False" w215 {
                              tunnel: w216 -> [w220 w233]
                              tunnel: [w219 w230] -> w205
                              tunnel: w214 -> [w218 _]
                              tunnel: w212 -> [w217 _]
                              frame False {
                                n112 = flat-sequence {
                                tunnel: w220 -> [w225]
                                tunnel: [w226] -> w221
                                tunnel: w218 -> [w226]
                                tunnel: w217 -> [w222]
                                tunnel: w221 -> [w228]
                                tunnel: [w227] -> w219
                                frame #0 {
                                n113 = control-ref of="Objective Running"() -> (w223:refnum<vi>)
                                n114 = call "ESA-C Move Axis To.vi"("Drive Connection Settings"=w226, "Axis"=1, "Current Voltage (V)"=w222, "Drive New Abs. Positions"=w225, "Running"=w223) -> ()  [unwired: 2 in]
                                }
                                frame #1 {
                                n115 = call "ESA-C Get Values.vi"("Drive Connection Settings"=w228) -> ("Drive Current Values"=w227:T1)
                                }
                                }
                              }
                              frame True {
                                n116 = Unbundle By Name(w233) -> ("Drive X Set"=w234:dbl, "Drive Y Set"=w231:dbl)
                                n117 = Wait (ms)(milliseconds to wait=u32 1000 ("Zu wartende ms")) -> ()  [unwired: 1 out]
                                n118 = Bundle By Name(cluster=T1 {"Voltages"={"Drive X Voltage"=0.0, "Drive Y Voltage"=0.0, "Drive Z Voltage"=0.0}, "Position"={"Drive X Position"=0.0, "Drive Y Position"=0.0, "Drive Z Position"=0.0}} ("Drive Current Values"), "Position.Drive X Position"=w234, "Position.Drive Y Position"=w231) -> (w230:T1)
                              }
                            }
                            n119 = global write "Global Variables.vi" "Global Drive Position"(w205) -> ()
                            n120 = local write "Current Position"(w205) -> ()
                            n121 = Unbundle By Name(w205) -> ("Position.Drive X Position"=w209:dbl, "Position.Drive Y Position"=w208:dbl)
                            n122 = Build Array (concatenate)(w210, w208) -> (w207:dbl[])
                            n123 = Build Array (concatenate)(w211, w209) -> (w206:dbl[])
                          }
                          frame #3 {
                            # "run measurement"
                            n124 = case shown="True" w239 {
                              tunnel: w250 -> [_ _]
                              tunnel: w249 -> [w257 w278]
                              tunnel: w248 -> [w256 w277]
                              tunnel: w247 -> [w259 w275]
                              tunnel: w246 -> [w260 w276]
                              tunnel: [w254 w272] -> w245
                              tunnel: [w255 w271] -> w244
                              tunnel: [w259 w274] -> w243
                              tunnel: [w260 w273] -> w242
                              tunnel: w241 -> [_ w280]
                              tunnel: w240 -> [_ w279]
                              tunnel: w238 -> [_ w268]
                              tunnel: w237 -> [_ w267]
                              tunnel: w236 -> [_ w265]
                              tunnel: w235 -> [_ w261]
                              frame False {
                                # "video mode (take snapshot)"
                                n125 = local read "Current Position"() -> (w258:T1)
                                n126 = Unbundle By Name(w258) -> ("Position.Drive X Position"=w253:dbl, "Position.Drive Y Position"=w252:dbl)
                                n127 = Build Array (concatenate)(w257, w253) -> (w254:dbl[])
                                n128 = Build Array (concatenate)(w256, w252) -> (w255:dbl[])
                                n129 = Build Array(w254, w255) -> (w251:dbl[][])
                                n130 = call "Video Snapshot.vi"() -> ()  [unwired: 11 in, 1 out]
                                n131 = local write "Live Data"(w251) -> ()
                              }
                              frame True {
                                # "spectra mode"
                                n132 = Unbundle By Name(w267) -> ("Repetitions"=w266:u16)
                                n133 = case shown="False" w279 {
                                tunnel: [w284 w303] -> w264
                                tunnel: w268 -> [w285 _]
                                tunnel: w266 -> [w283 _]
                                tunnel: w265 -> [w282 _]
                                frame False {
                                n134 = for {
                                N: w283 -> [w287]
                                shift-right: [w299] -> _
                                shift-left: w282 -> [w300]
                                tunnel: [w297] -> w284
                                tunnel: w285 -> [w295]
                                i -> [w302]
                                stop <- w294 continue-if-true
                                n135 = Number To Decimal String(number=w287) -> (decimal integer string=w290:string)  [unwired: 1 in]
                                n136 = control-ref of="CCD Running"() -> (w293:refnum<vi>)
                                n137 = control-ref of="Start"() -> (w292:refnum<vi>)
                                n138 = call "CCD3000 Spectral Acquisition.vi"("Acquire"=w292, "Running"=w293, "Comm Params"=w295) -> ("Raw-Spectrum"=w301:u16[])  [unwired: 6 in, 2 out]
                                n139 = local read "Wavelengths (nm)"() -> (w296:dbl[])
                                n140 = Build Array (concatenate)(w301, w300) -> (w299:u16[][])
                                n141 = Increment(x=w302) -> (x+1=w286:i32)
                                n142 = Number To Decimal String(number=w286) -> (decimal integer string=w289:string)  [unwired: 1 in]
                                n143 = Concatenate Strings(w289, "/" ("string"), w290) -> (w288:string)
                                n144 = local write "CCD3000 Current Rep."(w288) -> ()
                                n145 = local read "Start"() -> (w294:bool)
                                n146 = call "CCD3000 Average Spectra.vi"("Repetitions"=w286, "Raw Spectra"=w299) -> ("Raw Spectrum"=w298:dbl[])
                                n147 = call "CCD3000 Pixel to Wavelength v10.1.0.vi"("Wavelengths (nm)"=w296, "Raw Spectrum"=w298) -> ("Spectrum-Cluster"=w297:T14)  [unwired: 1 out]
                                }
                                }
                                frame True {
                                # "simulate spectrum"
                                n148 = call "Mapping Simulated Spectrum v10.1.0.vi"() -> ("Simulated Spectrum"=w303:cluster{i32[], dbl[]}[])
                                }
                                }
                                n149 = local read "Target Position"() -> (w270:T2)
                                n150 = Index Array(array=w264, index=0 ("Index")) -> (element=w263:T15)
                                n151 = call "Mapping Merge Live Data v10.2.1.vi"("New Spectrum"=w263, "Target Position"=w270, "X in (1D)"=w278, "Y in (1D)"=w277, "L in (2D)"=w276, "I in (2D)"=w275, "Step Size"=w261) -> ("Live Data"=w269:dbl[][], "X out (1D)"=w272:dbl[], "Y out (1D)"=w271:dbl[], "L out (2D)"=w273:dbl[][], "I out (2D)"=w274:dbl[][])  [unwired: 4 in]
                                n152 = invoke class="VI Interface Type 0" method="Ctrl Val.Set"(reference=w280, "Control Name"="LiveData" ("Elementname"), "Value"=w269) -> ()  [unwired: 2 in, 5 out]
                                n153 = local write "Live Data"(w269) -> ()
                              }
                            }
                          }
                          frame #4 {
                            # "set new X"
                            n154 = Increment(x=w314) -> (x+1=w313:i32)
                            n155 = local read "Start"() -> (w307:bool)
                            n156 = Equal?(x=w312, y=w313) -> (x = y?=w304:bool)
                            n157 = Not(x=w307) -> (.not. x?=w306:bool)
                            n158 = Or(x=w304, y=w306) -> (x .or. y?=w305:bool)
                            n159 = case shown="False" w305 {
                              tunnel: w311 -> [w322 w330]
                              tunnel: [w321 w330] -> w308
                              tunnel: w310 -> [w320 _]
                              tunnel: w309 -> [w315 _]
                              frame False {
                                n160 = Unbundle By Name(w322) -> ("Drive X Set"=w323:dbl)
                                n161 = case shown="False" w320 {
                                tunnel: w323 -> [w326 w328]
                                tunnel: [w325 w329] -> w316
                                tunnel: w315 -> [w324 w327]
                                frame False {
                                n162 = Subtract(x=w326, y=w324) -> (x-y=w325:dbl)
                                }
                                frame True {
                                n163 = Add(x=w328, y=w327) -> (x+y=w329:dbl)
                                }
                                }
                                n164 = Divide(x=w316, y=w315) -> (x/y=w319:dbl)
                                n165 = Round To Nearest(number=w319) -> (nearest integer value=w318:dbl)
                                n166 = Multiply(x=w318, y=w315) -> (x*y=w317:dbl)
                                n167 = Bundle By Name(cluster=w322, "Drive X Set"=w317) -> (w321:T13)
                              }
                              frame True {
                              }
                            }
                            n168 = local write "Target Position"(w308) -> ()
                          }
                          frame #5 {
                            n169 = Tick Count (ms)() -> (millisecond timer value=w335:u32)
                            n170 = Subtract(x=w335, y=w334) -> (x-y=w337:u32)
                            n171 = Divide(x=w337, y=u32 1000) -> (x/y=w332:dbl)
                            n172 = Build Array (concatenate)(w333, w332) -> (w331:dbl[])
                          }
                        }
                        n173 = local read "Start"() -> (w190:bool)
                      }
                    }
                    frame #1 {
                      # "set new Y\nand move to new position"
                      n174 = Increment(x=w349) -> (x+1=w348:i32)
                      n175 = local read "Start"() -> (w339:bool)
                      n176 = Equal?(x=w347, y=w348) -> (x = y?=w341:bool)
                      n177 = local read "Simulate Drive"() -> (w342:bool)
                      n178 = Not(x=w339) -> (.not. x?=w340:bool)
                      n179 = Or(x=w341, y=w340) -> (x .or. y?=w338:bool)
                      n180 = case shown="False" w338 {
                        tunnel: w345 -> [w370 w371]
                        tunnel: [w369 w371] -> w343
                        tunnel: w346 -> [w364 _]
                        frame False {
                          n181 = Unbundle By Name(w370) -> ("Drive Y Set"=w368:dbl)
                          n182 = Add(x=w364, y=w368) -> (x+y=w365:dbl)
                          n183 = Divide(x=w365, y=w364) -> (x/y=w366:dbl)
                          n184 = Round To Nearest(number=w366) -> (nearest integer value=w367:dbl)
                          n185 = Multiply(x=w367, y=w364) -> (x*y=w363:dbl)
                          n186 = Bundle By Name(cluster=w370, "Drive Y Set"=w363) -> (w369:T13)
                        }
                        frame True {
                        }
                      }
                      n187 = case shown="False" w342 {
                        tunnel: w344 -> [w354 _]
                        tunnel: w343 -> [w353 _]
                        frame False {
                          n188 = local read "Current Position"() -> (w352:T1)
                          n189 = Unbundle By Name(w352) -> ("Voltages.Drive Y Voltage"=w351:dbl)
                          n190 = flat-sequence {
                            tunnel: w354 -> [w356]
                            tunnel: w353 -> [w357]
                            tunnel: w351 -> [w358]
                            tunnel: [w356] -> w355
                            tunnel: [w362] -> w350
                            tunnel: w355 -> [w361]
                            frame #0 {
                              n191 = control-ref of="Objective Running"() -> (w360:refnum<vi>)
                              n192 = call "ESA-C Move Axis To.vi"("Drive Connection Settings"=w356, "Axis"=2, "Current Voltage (V)"=w358, "Drive New Abs. Positions"=w357, "Running"=w360) -> ()  [unwired: 2 in]
                            }
                            frame #1 {
                              n193 = call "ESA-C Get Values.vi"("Drive Connection Settings"=w361) -> ("Drive Current Values"=w362:T1)
                            }
                          }
                          n194 = global write "Global Variables.vi" "Global Drive Position"(w350) -> ()
                          n195 = local write "Current Position"(w350) -> ()
                        }
                        frame True {
                        }
                      }
                      n196 = local write "Target Position"(w343) -> ()
                    }
                  }
                  n197 = local read "Start"() -> (w133:bool)
                }
              }
              frame #2 {
                # "conclude measurement"
                n198 = flat-sequence {
                  tunnel: w373 -> [w381]
                  tunnel: w372 -> [w380]
                  tunnel: w374 -> [w389]
                  frame #0 {
                    # "save data"
                    n199 = global read "Global Variables.vi" "Global CCD Temperature (C)"() -> (w377:dbl)
                    n200 = global read "Global Variables.vi" "Global iHR Values"() -> (w375:T8)
                    n201 = local read "Mapping Params"() -> (w379:T5)
                    n202 = global read "Global Variables.vi" "Global ITC Values"() -> (w376:T7)
                    n203 = local read "Spectra Params"() -> (w384:T3)
                    n204 = Unbundle By Name(w379) -> ("Step Size"=w378:dbl)
                    n205 = local read "Live Data"() -> (w383:dbl[][])
                    n206 = call "Mapping Merge Real Positions v10.2.1.vi"("Live Data In"=w383, "X in (1D)"=w381, "Y in (1D)"=w380, "Step Size"=w378) -> ("Live Data Out"=w382:dbl[][])  [unwired: 11 in]
                    "Full Data" <- w382
                    n207 = call "Export_mappingFileName.vi"("ITC503 Current Values"=w376, "iHR Current Values"=w375, "Spectra Settings"=w384, "Mapping Parameters"=w379, "CCD3500 Temperature"=w377) -> ("Filename"=w385:string)
                    "Filename" <- w385
                    n208 = call "Export_2DtoTxt v10.2.0.vi"("Data (2D)"=w382, "Export Type"="Mapping", "Filename"=w385) -> ()  [unwired: 3 in]
                  }
                  frame #1 {
                    # "reset indicators"
                    n209 = case shown="False" w389 {
                      frame False {
                        n210 = call "Video Close.vi"() -> ()  [unwired: 11 in, 1 out]
                      }
                      frame True {
                      }
                    }
                    n211 = local write "Start"(FALSE ("Start")) -> ()
                    n212 = local write "CCD3000 Current Rep."("0/0" ("CCD3000 Current Rep.")) -> ()
                    n213 = global write "Global Variables.vi" "Mapping Running?"(FALSE ("Mapping Running?")) -> ()
                    n214 = property on="Measuring" class="Bool (strict)"("BoolText.Text"="" ("Boolescher Text.Text")) -> ()  [unwired: 2 in, 2 out]
                    n215 = property on="Measuring" class="Bool (strict)"("Blinking"=FALSE ("Measuring")) -> ()  [unwired: 2 in, 2 out]
                  }
                }
              }
            }
          }
        }
        n216 = local read "Exit"() -> (w40:bool)
      }
    }
    frame #2 {
      n217 = invoke class="VI Interface Type 0" method="Ctrl Val.Set"(reference=w394, "Control Name"="Exit" ("Elementname"), "Value"=TRUE) -> ()  [unwired: 2 in, 5 out]
      n218 = local read "AutoClose"() -> (w393:bool)
      n219 = flat-sequence {
        tunnel: w393 -> [w397]
        frame #0 {
          # "reset and close"
          n220 = control-ref of="Dieses VI"() -> (w400:refnum<vi>)
          n221 = global write "Global Variables.vi" "Mapping Open?"(FALSE ("Mapping Open?")) -> ()
          n222 = invoke class="VI" method="Default Vals.Reinit All"(reference=w400) -> (reference out=w398:refnum<vi>)  [unwired: 2 in, 2 out]
          n223 = property on="Measuring" class="Bool (strict)"("BoolText.Text"="" ("Boolescher Text.Text")) -> ()  [unwired: 2 in, 2 out]
          n224 = property class="App"() -> ("App.Kind"=w401:T16)  [unwired: 2 in, 2 out]
          n225 = case shown="\"Development System\"" w401 {
            tunnel: w398 -> [w403 w405]
            tunnel: w397 -> [_ w404]
            frame "invalid app kind", Default {
              n226 = invoke on="Invoke Node" class="VI" method="FP.Close"(reference=w403) -> ()  [unwired: 2 in, 3 out]
            }
            frame "Development System" {
              n227 = case shown="True" w404 {
                tunnel: w405 -> [_ w406]
                frame False {
                }
                frame True {
                  n228 = invoke on="Invoke Node" class="VI" method="FP.Close"(reference=w406) -> ()  [unwired: 2 in, 3 out]
                }
              }
            }
          }
        }
      }
    }
  }
